vi "Construct.vi"(8 "error in (no error)":errorcluster, 10 "SkipIfNotPresent?":bool=TRUE, 11 "MicronCLI":path=path "micronCLI.exe") -> (0 "error out":errorcluster, 2 "Present?":bool, 3 "MicronCLI out":refnum<class "MicronCLI.lvclass">)   [LabVIEW 2019, in "MicronCLI.lvclass"]
uses:
  MicronCLI.lvclass
  MicronCLI.lvclass/MicronCLI.ctl
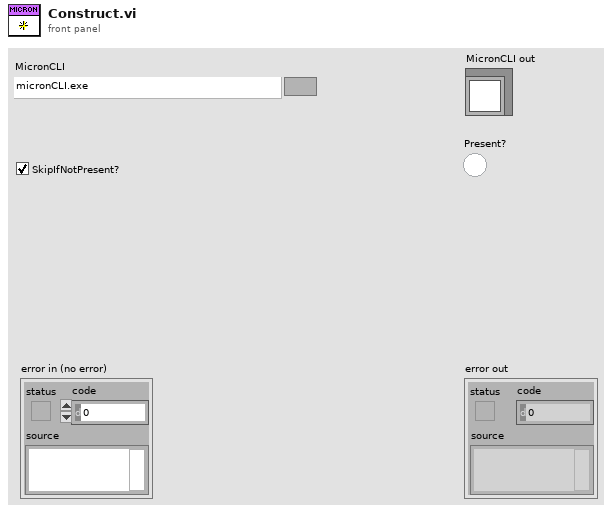
[diagram p1: front panel]
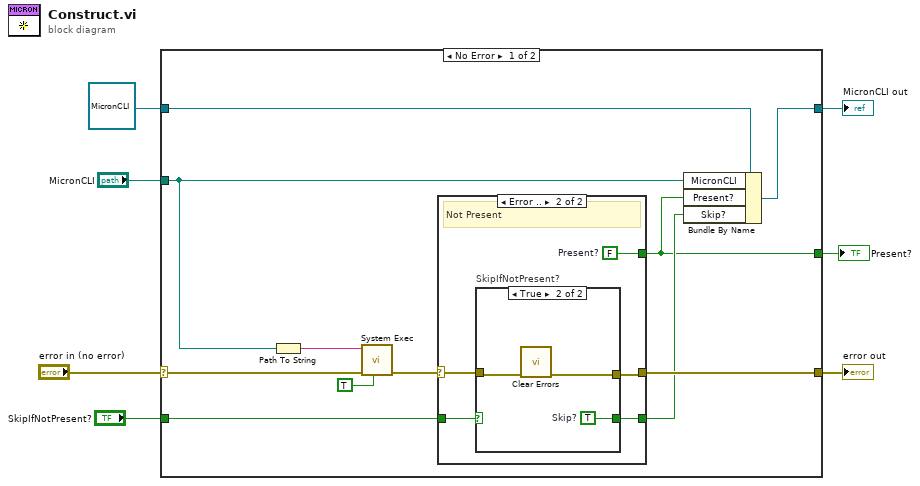
[diagram p0: block diagram]
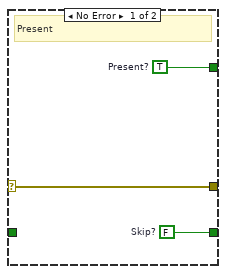
[diagram p2: hidden frame]
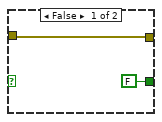
[diagram p3: hidden frame]
diagram:
  n1 = case shown="No Error" "error in (no error)" {
    selector: "error in (no error)" -> [w13 w33]
    tunnel: [w11 w33] -> w6
    tunnel: [w17 w32] -> w5
    tunnel: refnum<class "MicronCLI.lvclass"> refnum ("MicronCLI in") -> [w18 w32]
    tunnel: "MicronCLI" -> [w16 _]
    tunnel: "SkipIfNotPresent?" -> [w9 _]
    tunnel: [w8 _] -> w1
    frame No Error {
      n2 = Path To String(path=w16) -> (string=w14:string)
      n3 = call <vilib>:"System Exec.vi"("run minimized? (F)"=TRUE, "error in (no error)"=w13, "command line"=w14) -> ("error out"=w12:errorcluster)  [unwired: 5 in, 3 out]
      n4 = case shown="Error .." w12 {
        selector: w12 -> [w21 w24]
        tunnel: [w21 w23] -> w11
        tunnel: [w20 w26] -> w8
        tunnel: [w19 w22] -> w10
        tunnel: w9 -> [_ w25]
        frame No Error {
          w19 = FALSE  # Skip?
          w20 = TRUE  # Present?
          # "Present"
        }
        frame Error {
          w26 = FALSE  # Present?
          # "Not Present"
          n5 = case "SkipIfNotPresent?" shown="True" w25 {
            tunnel: w24 -> [w28 w31]
            tunnel: [w28 w30] -> w23
            tunnel: [FALSE w29] -> w22
            frame False {
            }
            frame True {
              w29 = TRUE  # Skip?
              n6 = call <vilib>:"Clear Errors.vi"("error in (no error)"=w31) -> ("error out"=w30:errorcluster)  [unwired: 5 in, 1 out]
            }
          }
        }
      }
      n7 = Bundle By Name(cluster=w18, "MicronCLI"=w16, "Present?"=w8, "Skip?"=w10) -> (w17:refnum<class "MicronCLI.lvclass">)
    }
    frame Error {
    }
  }
  "error out" <- w6
  "MicronCLI out" <- w5
  "Present?" <- w1
